vi "API get platform statue.vi"(9 "platformStatue input":i32[](array[numeric]), 11 "PlatformNum":i32) -> (1 "platformStatue output":i32[](array[numeric]), 3 "platformstatue return value":bool)   [LabVIEW 2011, in "API DYM.lvlib"]
uses:
  API DYM.lvlib
  DyMechnicalPlatform.dll
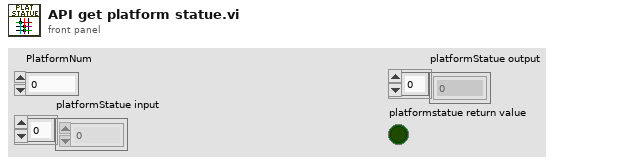
[diagram p1: front panel]
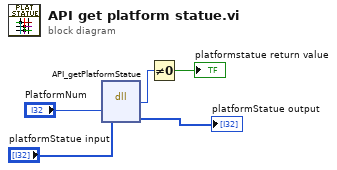
[diagram p0: block diagram]
diagram:
  n1 = dll-call lib="PTH1Xabs D可重构机电平台项目DemoLabViewDYSYSAPIDyMechnicalPlatform.dll" fn="API_getPlatformStatue"("PlatformNum"="PlatformNum", "platformStatue"="platformStatue input") -> ("PlatformStatue return value"=w2:i32, "platformStatue"=→"platformStatue output":i32[])  [unwired: 4 in, 2 out]
  n2 = Not Equal To 0?(x=w2) -> (x != 0?=→"platformstatue return value":bool)
